vi "Position Find Drone Button.vi"(8 "error in (no error) 2":errorcluster, 11 "Find Drone button":refnum<vi>) -> (0 "error out":errorcluster)   [LabVIEW 2014]
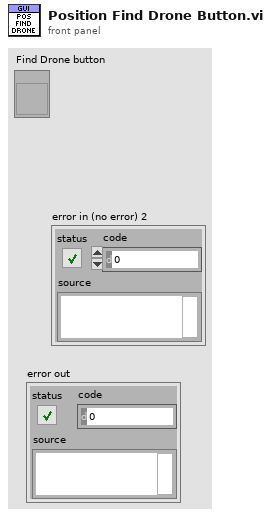
[diagram p1: front panel]
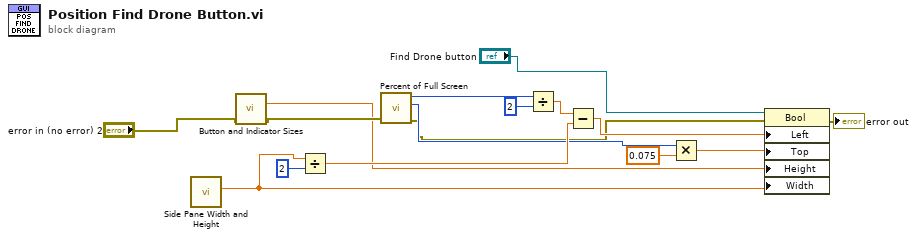
[diagram p0: block diagram]
diagram:
  n1 = call "Side Pane Width and Height.vi"() -> ("Width"=w6:dbl)  [unwired: 9 in, 2 out]
  n2 = call "Button and Indicator Sizes.vi"("error in (no error)"="error in (no error) 2") -> ("Button Height"=w7:dbl, "error out"=w8:errorcluster)  [unwired: 10 in, 3 out]
  n3 = Divide(x=w6, y=u32 2) -> (x/y=w12:dbl)
  n4 = call "Percent of Full Screen.vi"("error in (no error)"=w8) -> ("error out"=w2:errorcluster, "Bottom"=w4:i16, "Right"=w15:i16)  [unwired: 8 in]
  n5 = Divide(x=w15, y=i16 2) -> (x/y=w13:dbl)
  n6 = Subtract(x=w13, y=w12) -> (x-y=w11:dbl)
  n7 = Multiply(x=w4, y=0.075) -> (x*y=w3:dbl)
  n8 = property class="Bool"(reference="Find Drone button", error in=w2, "Left"=w11, "Top"=w3, "Height"=w7, "Width"=w6) -> (error out=→"error out":errorcluster)  [unwired: 1 out]
